vi "Update Target SV Tree.vi"(7 "TreeControl in":refnum<vi>, 8 "error in (no error)":errorcluster, 11 "Variable list compared":refnum<class "ChannelVS.lvclass">[](array[class])) -> (0 "error out":errorcluster)   [LabVIEW 2020, in "Shared Variables CD 2.0 Configuration.lvlib"]
uses:
  Shared Variables CD 2.0 Configuration.lvlib
  ChannelVS/ChannelVS.lvclass
  ChannelVS/ChannelVS.lvclass/ChannelVS.ctl
  built/windows/Channel.lvlibp/Channel.lvclass
  C:/Users/Administrator/Desktop/GIT/Shared-Variable-Custom-Device-2.0/Source/built/windows/Channel.lvlibp/Channel.lvclass
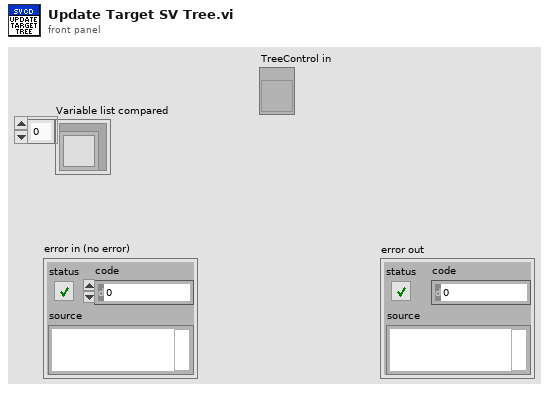
[diagram p1: front panel]
types:
  T1 = typedef "Channel.lvlibp/NI_Data Type.lvlib/Data Type.ctl" = enum8{"Invalid Type", "Void", "I8", "I16", "I32", "I64", "U8", "U16", "U32", "U64", "Single Float", "Double Float", "Extended Float", "Single Complex", "Double Complex", "Extended Complex", "Enum U8", "Enum U16", "Enum U32", "Enum U64", "Single Float With Unit", "Double Float With Unit", "Extended Float With Unit", "Single Complex with Unit", "Double Complex with Unit", "Extended Complex with Unit", "Boolean", "String", "Path", "Picture", "Tag", "Array", "Cluster", "Variant", "LV Variant", "Waveform", "Timestamp", "Digital Waveform", "Digital Data", "ExpressData", "Refnum", "External Data", "VI", "Poly VI", "LabVIEW Class Instance", "Fixed Point", "Set Collection", "Map Collection"}
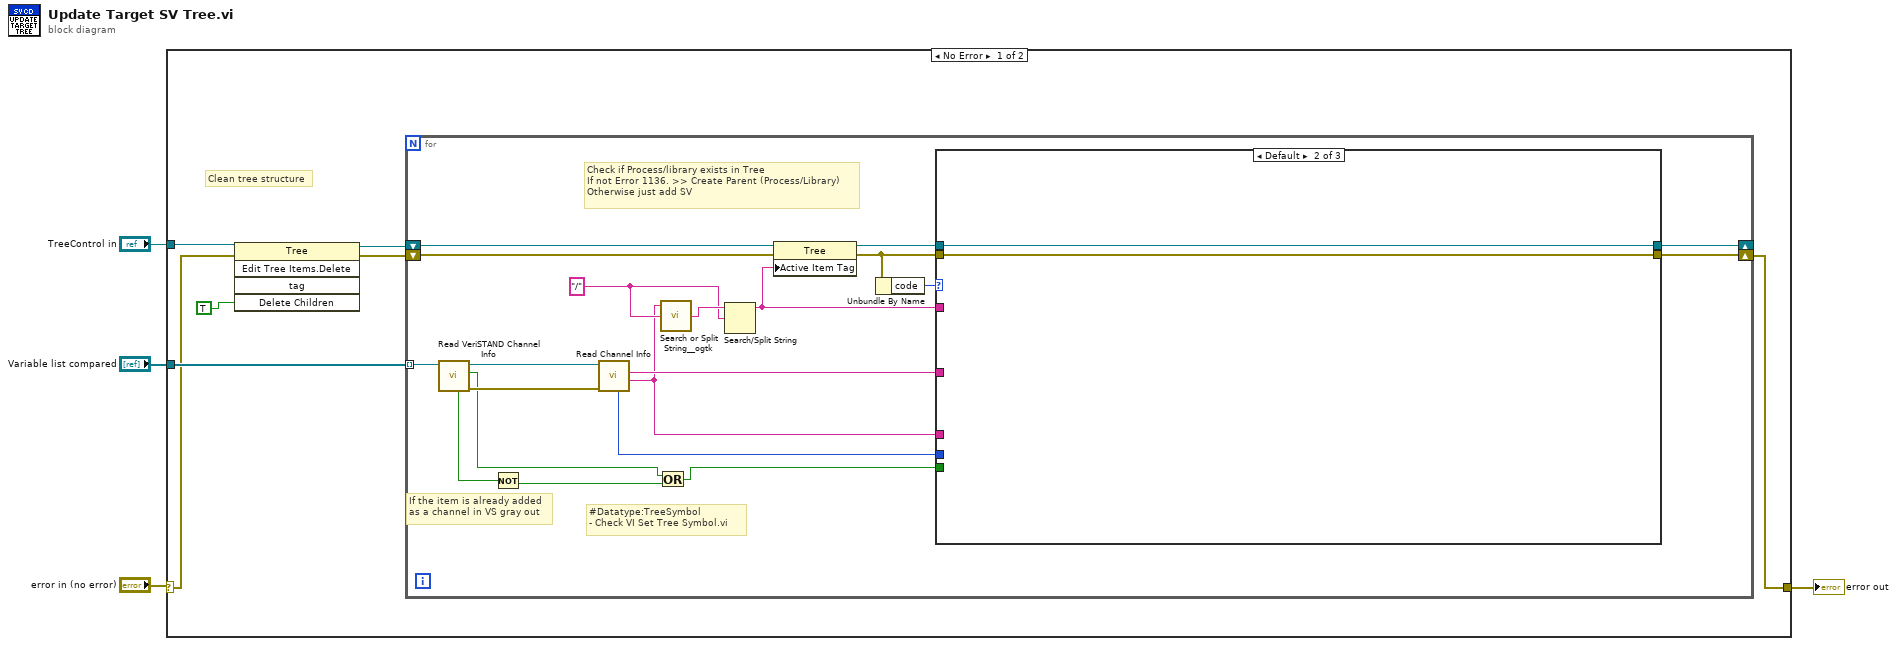
[diagram p0: block diagram]
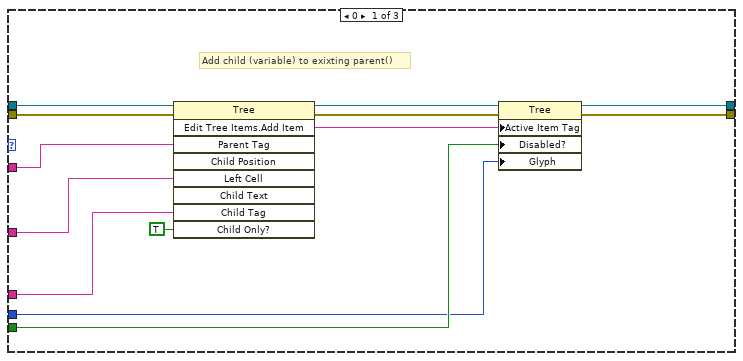
[diagram p2: hidden frame]
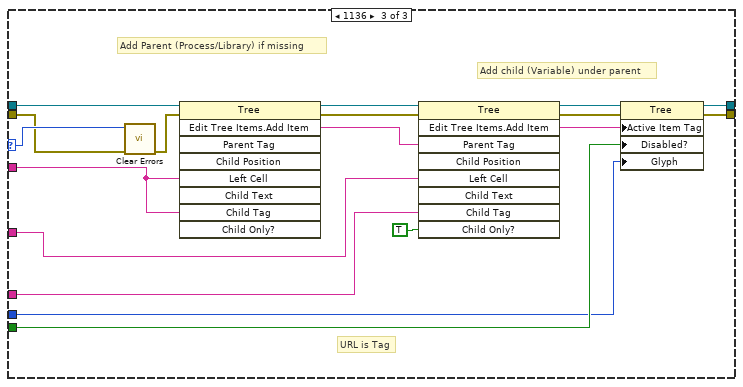
[diagram p3: hidden frame]
diagram:
  n1 = case shown="No Error" "error in (no error)" {
    selector: "error in (no error)" -> [w9 w65]
    tunnel: "TreeControl in" -> [w6 _]
    tunnel: "Variable list compared" -> [w11 _]
    tunnel: [w10 w65] -> w2
    frame No Error {
      # "Clean tree structure"
      n2 = invoke class="Tree" method="Edit Tree Items.Delete"(reference=w6, error in=w9, "Delete Children"=TRUE ("Delete Children?")) -> (reference out=w7:refnum<vi>, error out=w8:errorcluster)  [unwired: 2 in, 3 out]
      n3 = for {
        tunnel: w11 -> [w18] mode=indexing
        shift-right: [w23] -> _
        shift-left: w7 -> [w26]
        shift-right: [w22] -> w10
        shift-left: w8 -> [w25]
        w24 = "/" ("search string/char (-)")
        # "If the item is already added\nas a channel in VS gray out"
        # "#Datatype:TreeSymbol\n- Check VI Set Tree Symbol.vi"
        # "Check if Process/library exists in Tree \nIf not Error 1136. >> Create Parent (Process/Library)\nOtherwise just add SV"
        n4 = call "Read VeriSTAND Channel Info.vi"("ChannelVS in"=w18) -> ("error out"=w19:errorcluster, "Exist in VeriSTAND"=w14:bool, "ChannelVS out"=w17:refnum<class "ChannelVS.lvclass">, "Supported in CD"=w15:bool)  [unwired: 6 in, 1 out]
        n5 = Not(x=w15) -> (.not. x?=w13:bool)
        n6 = call "Read Channel Info.vi"("error in (no error)"=w19, "Channel in"=w17) -> ("URL"=w16:string, "Name"=w21:string, "DataType"=w20:T1)  [unwired: 4 in, 3 out]
        n7 = Or(x=w14, y=w13) -> (x .or. y?=w12:bool)
        n8 = call <userlib>:"Search or Split String__ogtk.vi"("search string/char (-)"=w24, "string"=w16) -> ("substring after match"=w31:string)  [unwired: 1 in, 2 out]
        n9 = Search/Split String(string=w31, search string/char (-)=w24) -> (substring before match=w27:string)  [unwired: 1 in, 2 out]
        n10 = property class="Tree"(reference=w26, error in=w25, "Active Item Tag"=w27) -> (reference out=w29:refnum<vi>, error out=w28:errorcluster)
        n11 = Unbundle By Name(w28) -> ("code"=w30:i32)
        n12 = case shown="Default" w30 {
          selector: w30 -> [_ _ w59]
          tunnel: w16 -> [w38 _ w55]
          tunnel: w27 -> [w44 _ w63]
          tunnel: w29 -> [w43 w46 w64]
          tunnel: w28 -> [w42 w45 w58]
          tunnel: [w36 w45 w51] -> w22
          tunnel: [w37 w46 w53] -> w23
          tunnel: w21 -> [w41 _ w56]
          tunnel: w12 -> [w34 _ w49]
          tunnel: w20 -> [w33 _ w48]
          frame 0 {
            # "Add child (variable) to exixting parent()"
            n13 = invoke on="Invoke Node" class="Tree" method="Edit Tree Items.Add Item"(reference=w43, error in=w42, "Parent Tag"=w44, "Left Cell"=w41, "Child Tag"=w38, "Child Only?"=TRUE) -> (reference out=w40:refnum<vi>, error out=w39:errorcluster, "Edit Tree Items:Add Item"=w32:string)  [unwired: 3 in, 6 out]
            n14 = property class="Tree"(reference=w40, error in=w39, "Active Item Tag"=w32, "Disabled?"=w34, "Glyph"=w33) -> (reference out=w37:refnum<vi>, error out=w36:errorcluster)
          }
          frame Default {
          }
          frame 1136 {
            # "Add child (Variable) under parent"
            # "Add Parent (Process/Library) if missing"
            # "URL is Tag"
            n15 = call <vilib>:"Clear Errors.vi"("error in (no error)"=w58, "specific error code to clear (0: all)"=w59) -> ("error out"=w57:errorcluster)  [unwired: 4 in, 1 out]
            n16 = invoke class="Tree" method="Edit Tree Items.Add Item"(reference=w64, error in=w57, "Left Cell"=w63, "Child Tag"=w63) -> (reference out=w62:refnum<vi>, error out=w61:errorcluster, "Edit Tree Items:Add Item"=w60:string)  [unwired: 5 in, 6 out]
            n17 = invoke on="Invoke Node" class="Tree" method="Edit Tree Items.Add Item"(reference=w62, error in=w61, "Parent Tag"=w60, "Left Cell"=w56, "Child Tag"=w55, "Child Only?"=TRUE) -> (reference out=w54:refnum<vi>, error out=w52:errorcluster, "Edit Tree Items:Add Item"=w47:string)  [unwired: 3 in, 6 out]
            n18 = property class="Tree"(reference=w54, error in=w52, "Active Item Tag"=w47, "Disabled?"=w49, "Glyph"=w48) -> (reference out=w53:refnum<vi>, error out=w51:errorcluster)
          }
        }
      }
    }
    frame Error {
    }
  }
  "error out" <- w2
